vi "read build root directory.vi"(11 "Builder in":refnum<class "Builder.lvclass">) -> (2 "build root directory":path)   [LabVIEW 2024, in "Builder.lvclass"]
uses:
  Builder.lvclass
  Builder.lvclass/Builder.ctl
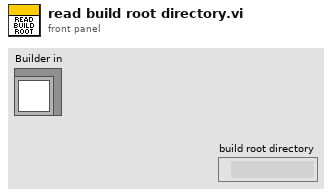
[diagram p1: front panel]
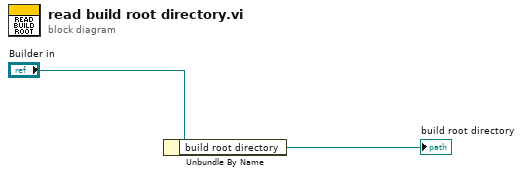
[diagram p0: block diagram]
diagram:
  n1 = Unbundle By Name("Builder in") -> ("build root directory"=→"build root directory":path)
